vi "princess.vi"   [LabVIEW 2015]
types:
  T1 = typedef "imagedata.ctl" = cluster{"image type":i32, "image depth":i32, "image":u8[], "mask":u8[], "colors":u32[], "Rectangle":cluster{"left":i16, "top":i16, "right":i16, "bottom":i16}}
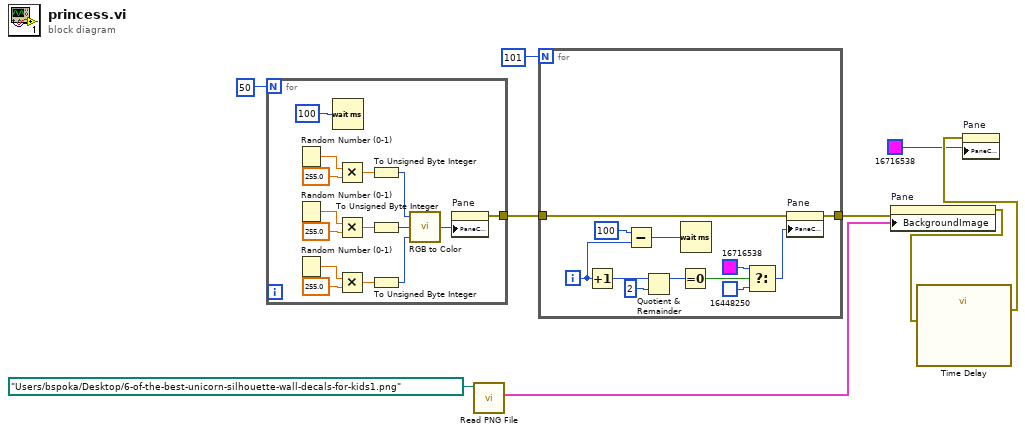
[diagram p0: block diagram]
diagram:
  n1 = for {
    N: 50 -> [_]
    tunnel: [w10] -> w7
    n2 = Random Number (0-1)() -> (number: 0 to 1=w24:dbl)
    n3 = Random Number (0-1)() -> (number: 0 to 1=w21:dbl)
    n4 = Random Number (0-1)() -> (number: 0 to 1=w18:dbl)
    n5 = Wait (ms)(milliseconds to wait=u32 100) -> ()  [unwired: 1 out]
    n6 = Multiply(x=w24, y=255.0) -> (x*y=w22:dbl)
    n7 = Multiply(x=w21, y=255.0) -> (x*y=w19:dbl)
    n8 = Multiply(x=w18, y=255.0) -> (x*y=w16:dbl)
    n9 = To Unsigned Byte Integer(number=w22) -> (unsigned 8bit integer=w15:u8)
    n10 = To Unsigned Byte Integer(number=w19) -> (unsigned 8bit integer=w14:u8)
    n11 = To Unsigned Byte Integer(number=w16) -> (unsigned 8bit integer=w13:u8)
    n12 = call <vilib>:"RGB to Color.vi"("B"=w13, "G"=w14, "R"=w15) -> ("Color"=w12:u32)
    n13 = property on="Pane" class="Pane"("PaneColor"=w12) -> (error out=w10:errorcluster)  [unwired: 2 in, 1 out]
  }
  n14 = call <vilib>:"Read PNG File.vi"("path to PNG file"=path "/Users/bspoka/Desktop/6-of-the-best-unicorn-silhouette-wall-decals-for-kids1.png") -> ("image data"=w5:T1)  [unwired: 8 in, 2 out]
  n15 = for {
    N: 101 -> [_]
    tunnel: w7 -> [w31]
    tunnel: [w25] -> w4
    i -> [w27]
    n16 = Increment(x=w27) -> (x+1=w35:i32)
    n17 = Subtract(x=u32 100 ("milliseconds to wait"), y=w27) -> (x-y=w26:u32)
    n18 = Quotient & Remainder(x=w35, y=2) -> (x-y*floor(x/y)=w30:i32)  [unwired: 1 out]
    n19 = Equal To 0?(x=w30) -> (x = 0?=w29:bool)
    n20 = Wait (ms)(milliseconds to wait=w26) -> ()  [unwired: 1 out]
    n21 = Select(t=u32 16716538, s=w29, f=u32 16448250) -> (s? t:f=w32:u32)
    n22 = property on="Pane" class="Pane"(error in=w31, "PaneColor"=w32) -> (error out=w25:errorcluster)  [unwired: 1 in, 1 out]
  }
  n23 = property on="Pane" class="Pane"(error in=w4, "BackgroundImage"=w5) -> (error out=w3:errorcluster)  [unwired: 1 in, 1 out]
  n24 = call "Time Delay"("error in (no error)"=w3) -> ("error out"=w2:errorcluster)  [unwired: 10 in]
  n25 = property on="Pane" class="Pane"(error in=w2, "PaneColor"=u32 16716538) -> ()  [unwired: 1 in, 2 out]
